vi "Add manually search path.vi"(8 "error in (no error)":errorcluster, 11 "string in":string) -> (0 "error out":errorcluster, 1 "manual path out":string, 3 "cancelled?":bool)   [LabVIEW 2012, in "ServiceManager.lvclass"]
uses:
  ServiceManager.lvclass
panel:
  in  "button:cancel":bool
  in  "button:ok":bool
  in  "manual path":string
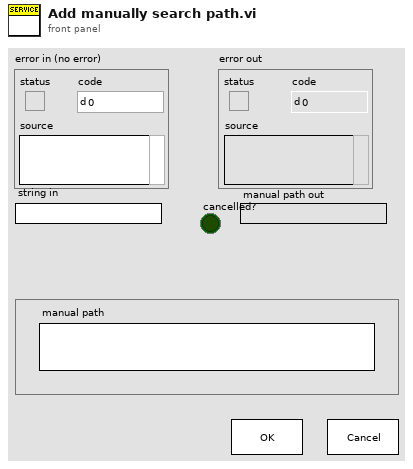
[diagram p1: front panel]
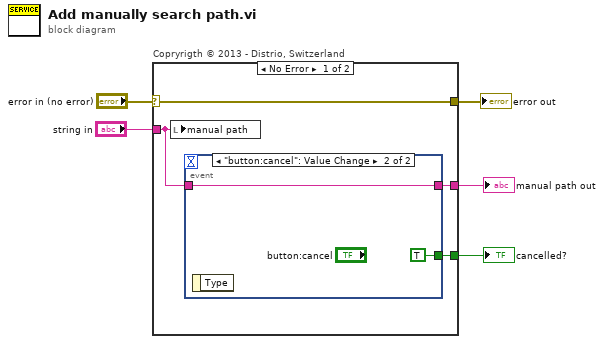
[diagram p0: block diagram]
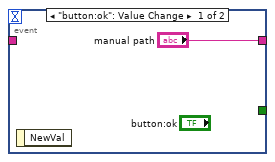
[diagram p2: hidden frame]
diagram:
  n1 = case "Copryrigth © 2013 - Distrio, Switzerland" shown="No Error" "error in (no error)" {
    selector: "error in (no error)" -> [w7 w13]
    tunnel: [w9 _] -> w5
    tunnel: [w8 _] -> w4
    tunnel: [w7 w13] -> w2
    tunnel: "string in" -> [w6 _]
    frame No Error {
      n2 = local write "manual path"(w6) -> ()
      n3 = event shown="[1] \"button:cancel\": Value Change" {
        selector: _ -> [_ _]
        dyn-events: _ -> [_ _]
        timeout: _ -> [_ _]
        tunnel: ["manual path" w11] -> w9
        tunnel: [_ TRUE ("button:cancel")] -> w8
        tunnel: w6 -> [_ w11]
        event "button:ok": Value Change {
          n4 = event-data() -> ()  [unwired: 1 in, 1 out]
        }
        event "button:cancel": Value Change {
          n5 = event-data() -> ()  [unwired: 1 in, 1 out]
        }
      }
    }
    frame Error {
    }
  }
  "manual path out" <- w5
  "cancelled?" <- w4
  "error out" <- w2
